vi "generate test config.vi"   [LabVIEW 2017, in "Data Sharing Framework System Explorer.lvlib"]
uses:
  Data Sharing Framework System Explorer.lvlib
  dsf core/Source/DSF Configuration API/1.0.0/DSF Configuration API.lvlib
  dsf core/Source/DSF Configuration API/1.0.0/Public/Controls/DSF Settings Info.ctl
  dsf core/Source/DSF Configuration API/1.0.0/Public/Controls/DSF Channel Info.ctl
  <userlib>/_OpenG.lib/numeric/numeric.llb/Random Number Within Range - I32__ogtk.vi
  dsf core/Source/DSF Configuration API/1.0.0/Public/Controls/DSF Transfer Info.ctl
  dsf core/Source/DSF Configuration API/1.0.0/Public/Write Item/Write Channel.vi
  dsf core/Source/DSF Configuration API/1.0.0/Public/Write Item/Write Settings.vi
  dsf core/Source/DSF Configuration API/1.0.0/Public/Write Item/Write Transfer.vi
  dsf core/Source/DSF Configuration API/1.0.0/Public/Write Item/Write Group.vi
  dsf core/Source/DSF Configuration API/1.0.0/Public/Controls/DSF Timing Info.ctl
  dsf core/Source/DSF Configuration API/1.0.0/Public/Controls/DSF Group Info.ctl
  dsf core/Source/DSF Configuration API/1.0.0/Public/Write Item/Write Plugin.vi
  dsf core/Source/DSF Configuration API/1.0.0/Public/Controls/DSF Plugin Info.ctl
  dsf core/Source/DSF Configuration API/1.0.0/Public/Controls/DSF Data Type.ctl
  dsf core/Source/DSF Configuration API/1.0.0/Public/Controls/DSF Byte Order.ctl
  dsf core/Source/DSF Configuration API/1.0.0/Public/Controls/DSF Direction.ctl
types:
  T1 = typedef "DSF Configuration API.lvlib/DSF Config Data RefNum.ctl" = refnum<k1>
  T2 = typedef "DSF Configuration API.lvlib/DSF Settings Info.ctl" = cluster{"key":string, "value":string}[]
  T3 = typedef "DSF Configuration API.lvlib/DSF Channel Info.ctl" = cluster{"count":u64, "buffer offset":u64, "data type":T4, "settings id":string}
  T4 = typedef "DSF Configuration API.lvlib/DSF Data Type.ctl" = enum8{"Bool", "SGL", "DBL", "I8", "I16", "I32", "I64", "U8", "U16", "U32", "U64"}
  T5 = typedef "DSF Configuration API.lvlib/DSF Transfer Info.ctl" = cluster{"byte order":T6, "channel ids":string[], "settings id":string}
  T6 = typedef "DSF Configuration API.lvlib/DSF Byte Order.ctl" = enum8{"big-endian", "little-endian"}
  T7 = typedef "DSF Configuration API.lvlib/DSF Group Info.ctl" = cluster{"direction":T8, "timing":T9, "transfer ids":string[], "settings id":string}
  T8 = typedef "DSF Configuration API.lvlib/DSF Direction.ctl" = enum8{"Tx", "Rx"}
  T9 = typedef "DSF Configuration API.lvlib/DSF Timing Info.ctl" = cluster{"priority":u64, "decimation":u64, "offset":u64}
  T10 = typedef "DSF Configuration API.lvlib/DSF Plugin Info.ctl" = cluster{"type":string, "timing":T9, "group ids":string[], "settings id":string}
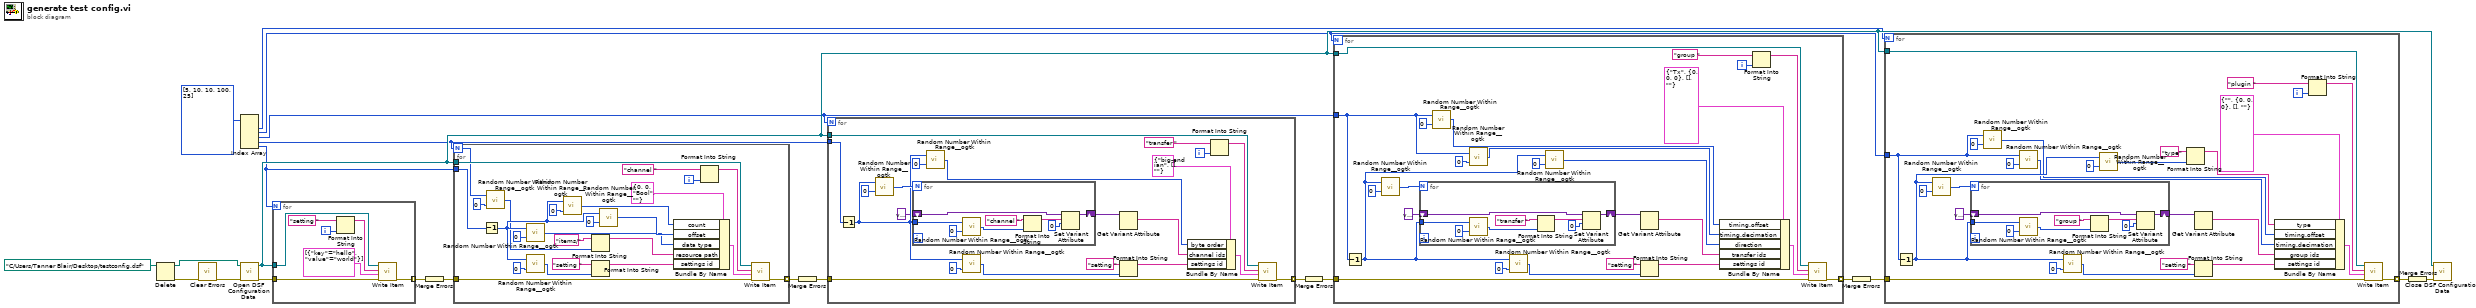
[diagram p0: block diagram]
diagram:
  n1 = Delete(path (use dialog)=path "C:/Users/Tanner Blair/Desktop/testconfig.dsf" ("configuration file path")) -> (deleted path=w3:path, error out=w2:errorcluster)  [unwired: 4 in, 1 out]
  n2 = call <vilib>:"Clear Errors.vi"("error in (no error)"=w2) -> ("error out"=w1:errorcluster)  [unwired: 5 in, 1 out]
  n3 = Index Array(array=i32[] [5, 10, 10, 100, 25]) -> (element #1=w8:i32, element #2=w4:i32, element #3=w5:i32, element #4=w6:i32, element #5=w7:i32)  [unwired: 5 in]
  n4 = call "Open DSF Configuration Data.vi"("error in (no error)"=w1, "dsf configuration file path"=w3) -> ("error out"=w21:errorcluster, "dsf refnum"=w14:T1)  [unwired: 5 in, 3 out]
  n5 = for {
    N: w7 -> [_]
    tunnel: w14 -> [w29]
    tunnel: w21 -> [w26]
    tunnel: [w25] -> w20 mode=indexing
    i -> [w28]
    n6 = Format Into String(initial string="setting ", w28) -> (resulting string=w23:string)  [unwired: 2 in, 1 out]
    n7 = call-poly "Write Item.vi"("error in (no error)"=w26, "settings values"=T2 [{"key"="hello", "value"="world"}], "id"=w23, "dsf refnum"=w29) -> ("error out"=w25:errorcluster)  [unwired: 5 in, 2 out]
  }
  n8 = Merge Errors(w20) -> (w19:errorcluster)
  n9 = for {
    N: w6 -> [w37]
    tunnel: w14 -> [w54]
    tunnel: w19 -> [w52]
    tunnel: [w51] -> w18 mode=indexing
    tunnel: w7 -> [w32]
    i -> [w53]
    n10 = Decrement(x=w32) -> (x-1=w41:i32)
    n11 = call-poly <userlib>:"Random Number Within Range__ogtk.vi"("High"=w37, "Low"=0) -> ("Random Number"=w35:i32)  [unwired: 3 in]
    n12 = call-poly <userlib>:"Random Number Within Range__ogtk.vi"("High"=w41, "Low"=0) -> ("Random Number"=w43:i32)  [unwired: 3 in]
    n13 = call-poly <userlib>:"Random Number Within Range__ogtk.vi"("High"=w41, "Low"=0) -> ("Random Number"=w40:i32)  [unwired: 3 in]
    n14 = call-poly <userlib>:"Random Number Within Range__ogtk.vi"("High"=w41, "Low"=0) -> ("Random Number"=w48:i32)  [unwired: 3 in]
    n15 = Format Into String(initial string="items/", w35) -> (resulting string=w34:string)  [unwired: 2 in, 1 out]
    n16 = Format Into String(initial string="setting ", w40) -> (resulting string=w39:string)  [unwired: 2 in, 1 out]
    n17 = call-poly <userlib>:"Random Number Within Range__ogtk.vi"("High"=w41, "Low"=0) -> ("Random Number"=w44:i32)  [unwired: 3 in]
    n18 = Bundle By Name(cluster=T3 {"count"=0, "buffer offset"=0, "data type"=enum."Bool", "settings id"=""} ("channel values"), "count"=w48, "offset"=w44, "data type"=w43, "resource path"=w34, "settings id"=w39) -> (w30:T3)
    n19 = Format Into String(initial string="channel ", w53) -> (resulting string=w31:string)  [unwired: 2 in, 1 out]
    n20 = call-poly "Write Item.vi"("error in (no error)"=w52, "channel values"=w30, "id"=w31, "dsf refnum"=w54) -> ("error out"=w51:errorcluster)  [unwired: 5 in, 2 out]
  }
  n21 = Merge Errors(w18) -> (w16:errorcluster)
  n22 = for {
    N: w5 -> [_]
    tunnel: w14 -> [w75]
    tunnel: w16 -> [w72]
    tunnel: [w71] -> w17 mode=indexing
    tunnel: w6 -> [w57]
    i -> [w74]
    n23 = Decrement(x=w57) -> (x-1=w61:i32)
    n24 = call-poly <userlib>:"Random Number Within Range__ogtk.vi"("High"=w61, "Low"=0) -> ("Random Number"=w62:i32)  [unwired: 3 in]
    n25 = for {
      N: w62 -> [_]
      tunnel: w61 -> [w82]
      shift-right: [w77] -> w59
      shift-left: variant ("Variant") -> [w81]
      n26 = call-poly <userlib>:"Random Number Within Range__ogtk.vi"("High"=w82, "Low"=0) -> ("Random Number"=w80:i32)  [unwired: 3 in]
      n27 = Format Into String(initial string="channel ", w80) -> (resulting string=w79:string)  [unwired: 2 in, 1 out]
      n28 = Set Variant Attribute(Variant=w81, name=w79, value=0 ("Low")) -> (Variant out=w77:variant)  [unwired: 1 in, 2 out]
    }
    n29 = call-poly <userlib>:"Random Number Within Range__ogtk.vi"("High"=w61, "Low"=0) -> ("Random Number"=w68:i32)  [unwired: 3 in]
    n30 = call-poly <userlib>:"Random Number Within Range__ogtk.vi"("High"=w61, "Low"=0) -> ("Random Number"=w64:i32)  [unwired: 3 in]
    n31 = Get Variant Attribute(Variant=w59) -> (names=w58:string[])  [unwired: 3 in, 3 out]
    n32 = Format Into String(initial string="setting ", w64) -> (resulting string=w63:string)  [unwired: 2 in, 1 out]
    n33 = Bundle By Name(cluster=T5 {"byte order"=enum."big-endian", "channel ids"=[], "settings id"=""} ("channel values"), "byte order"=w68, "channel ids"=w58, "settings id"=w63) -> (w56:T5)
    n34 = Format Into String(initial string="transfer ", w74) -> (resulting string=w55:string)  [unwired: 2 in, 1 out]
    n35 = call-poly "Write Item.vi"("error in (no error)"=w72, "transfer values"=w56, "id"=w55, "dsf refnum"=w75) -> ("error out"=w71:errorcluster)  [unwired: 5 in, 2 out]
  }
  n36 = Merge Errors(w17) -> (w15:errorcluster)
  n37 = for {
    N: w4 -> [_]
    tunnel: w14 -> [w108]
    tunnel: w15 -> [w105]
    tunnel: [w104] -> w13 mode=indexing
    tunnel: w5 -> [w86]
    i -> [w107]
    n38 = Decrement(x=w86) -> (x-1=w94:i32)
    n39 = call-poly <userlib>:"Random Number Within Range__ogtk.vi"("High"=w94, "Low"=0) -> ("Random Number"=w95:i32)  [unwired: 3 in]
    n40 = for {
      N: w95 -> [_]
      tunnel: w94 -> [w115]
      shift-right: [w110] -> w92
      shift-left: variant ("Variant") -> [w114]
      n41 = call-poly <userlib>:"Random Number Within Range__ogtk.vi"("High"=w115, "Low"=0) -> ("Random Number"=w113:i32)  [unwired: 3 in]
      n42 = Format Into String(initial string="transfer ", w113) -> (resulting string=w112:string)  [unwired: 2 in, 1 out]
      n43 = Set Variant Attribute(Variant=w114, name=w112, value=0 ("Low")) -> (Variant out=w110:variant)  [unwired: 1 in, 2 out]
    }
    n44 = call-poly <userlib>:"Random Number Within Range__ogtk.vi"("High"=w86, "Low"=0) -> ("Random Number"=w87:i32)  [unwired: 3 in]
    n45 = call-poly <userlib>:"Random Number Within Range__ogtk.vi"("High"=w86, "Low"=0) -> ("Random Number"=w88:i32)  [unwired: 3 in]
    n46 = call-poly <userlib>:"Random Number Within Range__ogtk.vi"("High"=w94, "Low"=0) -> ("Random Number"=w97:i32)  [unwired: 3 in]
    n47 = call-poly <userlib>:"Random Number Within Range__ogtk.vi"("High"=w94, "Low"=0) -> ("Random Number"=w101:i32)  [unwired: 3 in]
    n48 = Get Variant Attribute(Variant=w92) -> (names=w91:string[])  [unwired: 3 in, 3 out]
    n49 = Format Into String(initial string="setting ", w97) -> (resulting string=w96:string)  [unwired: 2 in, 1 out]
    n50 = Bundle By Name(cluster=T7 {"direction"=enum."Tx", "timing"={"priority"=0, "decimation"=0, "offset"=0}, "transfer ids"=[], "settings id"=""} ("channel values"), "timing.offset"=w87, "timing.decimation"=w88, "direction"=w101, "transfer ids"=w91, "settings id"=w96) -> (w85:T7)
    n51 = Format Into String(initial string="group ", w107) -> (resulting string=w84:string)  [unwired: 2 in, 1 out]
    n52 = call-poly "Write Item.vi"("error in (no error)"=w105, "group values"=w85, "id"=w84, "dsf refnum"=w108) -> ("error out"=w104:errorcluster)  [unwired: 5 in, 2 out]
  }
  n53 = Merge Errors(w13) -> (w12:errorcluster)
  n54 = for {
    N: w8 -> [_]
    tunnel: w14 -> [w143]
    tunnel: w12 -> [w140]
    tunnel: [w139] -> w11 mode=indexing
    tunnel: w4 -> [w119]
    i -> [w142]
    n55 = Decrement(x=w119) -> (x-1=w130:i32)
    n56 = call-poly <userlib>:"Random Number Within Range__ogtk.vi"("High"=w130, "Low"=0) -> ("Random Number"=w131:i32)  [unwired: 3 in]
    n57 = for {
      N: w131 -> [_]
      tunnel: w130 -> [w150]
      shift-right: [w145] -> w128
      shift-left: variant ("Variant") -> [w149]
      n58 = call-poly <userlib>:"Random Number Within Range__ogtk.vi"("High"=w150, "Low"=0) -> ("Random Number"=w148:i32)  [unwired: 3 in]
      n59 = Format Into String(initial string="group ", w148) -> (resulting string=w147:string)  [unwired: 2 in, 1 out]
      n60 = Set Variant Attribute(Variant=w149, name=w147, value=0 ("Low")) -> (Variant out=w145:variant)  [unwired: 1 in, 2 out]
    }
    n61 = call-poly <userlib>:"Random Number Within Range__ogtk.vi"("High"=w119, "Low"=0) -> ("Random Number"=w123:i32)  [unwired: 3 in]
    n62 = call-poly <userlib>:"Random Number Within Range__ogtk.vi"("High"=w119, "Low"=0) -> ("Random Number"=w124:i32)  [unwired: 3 in]
    n63 = call-poly <userlib>:"Random Number Within Range__ogtk.vi"("High"=w130, "Low"=0) -> ("Random Number"=w133:i32)  [unwired: 3 in]
    n64 = call-poly <userlib>:"Random Number Within Range__ogtk.vi"("High"=w130, "Low"=0) -> ("Random Number"=w122:i32)  [unwired: 3 in]
    n65 = Format Into String(initial string="type", w122) -> (resulting string=w120:string)  [unwired: 2 in, 1 out]
    n66 = Get Variant Attribute(Variant=w128) -> (names=w127:string[])  [unwired: 3 in, 3 out]
    n67 = Format Into String(initial string="setting ", w133) -> (resulting string=w132:string)  [unwired: 2 in, 1 out]
    n68 = Bundle By Name(cluster=T10 {"type"="", "timing"={"priority"=0, "decimation"=0, "offset"=0}, "group ids"=[], "settings id"=""} ("channel values"), "type"=w120, "timing.offset"=w123, "timing.decimation"=w124, "group ids"=w127, "settings id"=w132) -> (w118:T10)
    n69 = Format Into String(initial string="plugin ", w142) -> (resulting string=w117:string)  [unwired: 2 in, 1 out]
    n70 = call-poly "Write Item.vi"("error in (no error)"=w140, "plugin values"=w118, "id"=w117, "dsf refnum"=w143) -> ("error out"=w139:errorcluster)  [unwired: 5 in, 2 out]
  }
  n71 = Merge Errors(w11) -> (w10:errorcluster)
  n72 = call "Close DSF Configuration Data.vi"("error in (no error)"=w10, "dsf refnum"=w14) -> ()  [unwired: 8 in, 2 out]
